vi "Illini Hyperloop GUI v5.0.vi"() -> ()   [LabVIEW 2015]
uses:
  <vilib>/robotics/Controls/Attitude Indicator/Attitude Indicator.xctl
panel:
  out "Numeric 3":u16
  out "volat":dbl
  out "vy":dbl
  out "X2 Sen Stat":u16 format="%b"
  out "X1 Sen Stat":u16 format="%b"
  out "Tape Count":dbl
  out "Optical":dbl
  out "Temp5":dbl
  out "Temp4":dbl
  out "Temp3":dbl
  out "Temp2":dbl
  out "Temp1":dbl
  out "Time Since Coast":dbl
  out "Time Since Accel":dbl
  out "PCB Current mA":dbl(slide) scale=0.0..200.0
  out "Voltage 2":dbl(slide) scale=0.0..17.0
  out "True Position":dbl
  out "Sensor Status Bits":u16 format="%b"
  out "Pressure Status":bool
  out "Temp Status":bool=TRUE
  out "Velocity Status":bool
  out "Position Status":bool
  out "Acceleration Status":bool
  out "Voltage Status":bool
  out "PCB Current Status":bool
  in  "Pod State":u16(ring) items=["Pod Startup", "Safety Setup", "Safe Mode", "Functional Test", "Launch Ready", "Accel", "Coast", "Brake"]
  out "X2 Online":bool
  out "X1 Online":bool
  out "X2 State":dbl
  out "X1 State":dbl
  out "Position Chart":dbl(graph)
  out "Brake Pressure":dbl
  out "RPM":dbl
  out "Accel 3":dbl
  out "Accel 2":dbl
  out "Accel 1":dbl
  out "True Accel":dbl
  out "True Velocity":dbl
  out "Pull Tab connected":bool
  out "Voltage 1":dbl(slide) scale=0.0..17.0
  out "Ride Height":cluster{u16, u16, u16}(graph)
  out "Y, Z Accel":cluster{u16, u16}(graph)
  out "Temp Chart":cluster{u16, u16, u16, u16, u16}(graph)
  out "Brake Pressure Chart":dbl(graph)
  out "Velocity chart":dbl(graph)
  out "Acceleration Chart":cluster{dbl, dbl, dbl, dbl}(graph)
  in  "Send Command Button":bool
  in  "Command to Send":T1(ring)
  in  "Connection Status":enum16{"Disconnected", "Connected"}(ring)
  out "Attitude Indicator":cluster{"Roll":dbl, "Pitch":dbl}(xcontrol)
  in  "EMERGENCY BRAKE":bool
  in  "Functional Test Tab Control":enum32{"Network / File Info", "Program Control"}(tab)
  out "Client Closed":string="The client VI closed the connection."
  in  "Connect to":string="192.168.137.100"
  in  "timeout ms":i32=1000
  in  "port":u16=8800
  in  "ms per loop":u32
  in  "bytes per write":i32=1000
  out "Base File Name":string
  in  "Stop Program":bool
  out "Producer Error Messages":errorcluster
  out "Consumer Error Messages":errorcluster
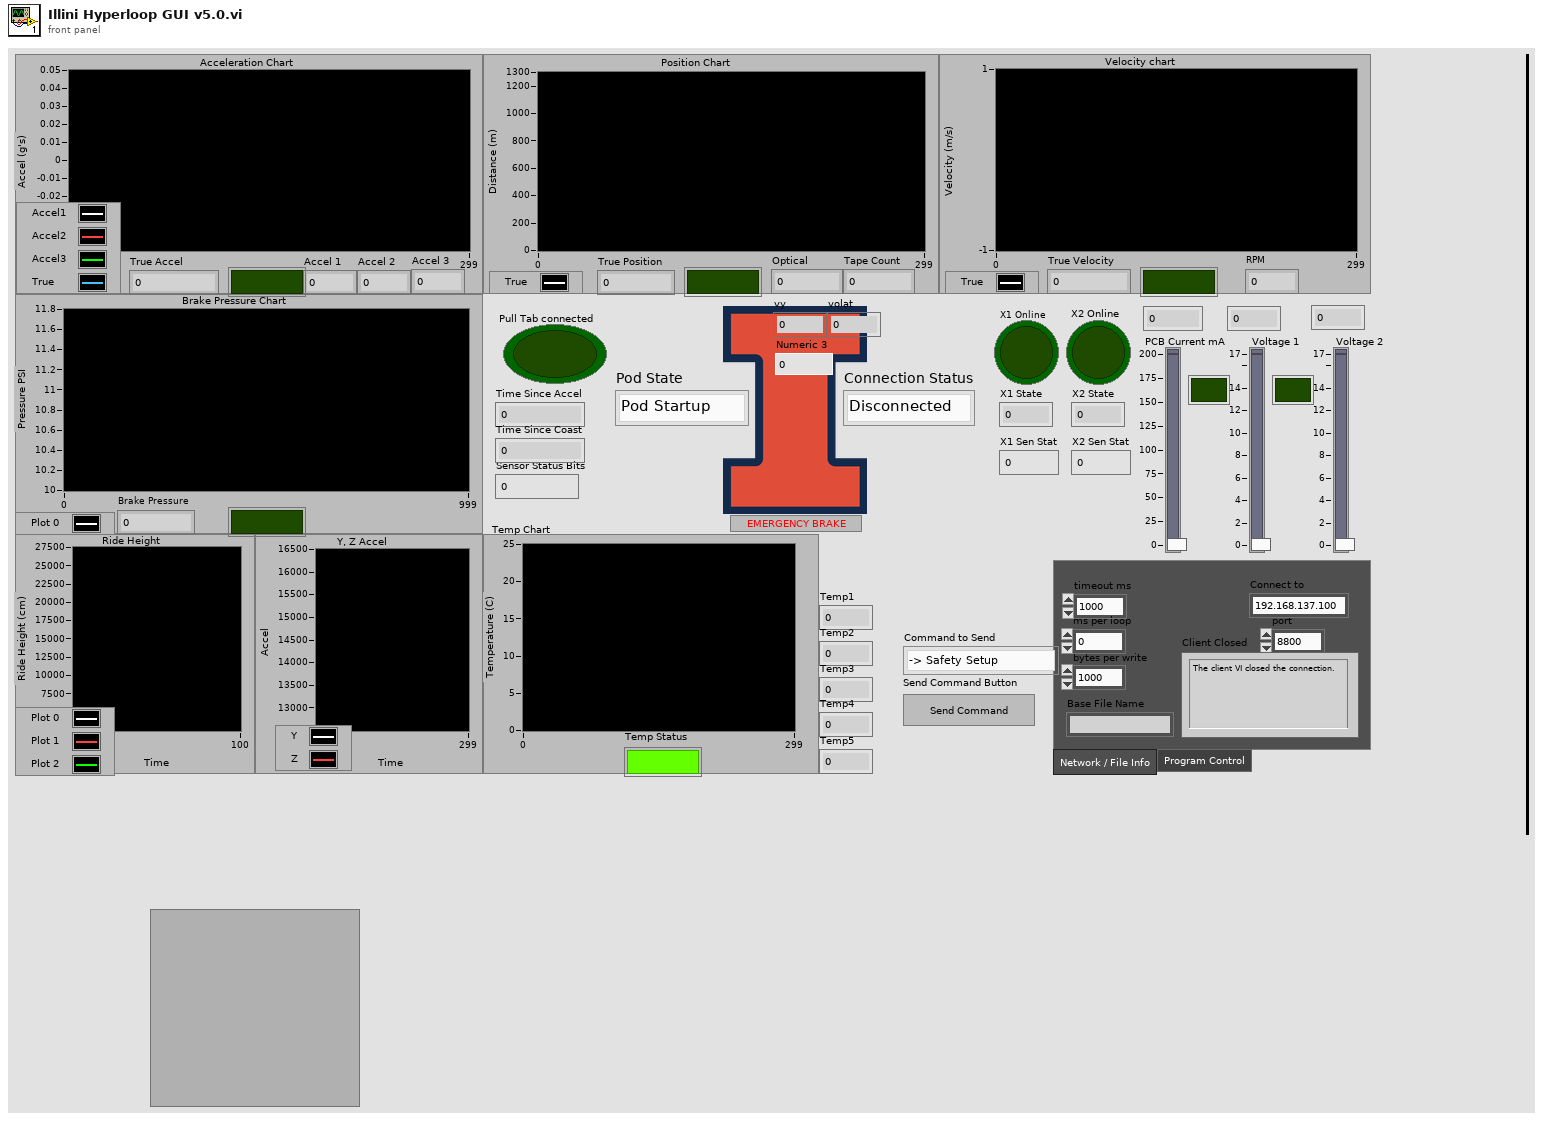
[diagram p1: front panel]
types:
  T1 = enum16{"-> Safety Setup", "-> Safe Mode", "-> Functional Test", "-> Ready to Launch", "-> Flight Brake", "EMERGENCY BRAKE", "Reset Sensors", "Calibrate Sensors", "Manual Brake ", "Manual Brake Reverse"}
  T2 = enum16{"Standard", "Buffered", "CRLF", "Immediate"}
  T3 = cluster{"Numeric 3":u16, "Numeric 3":u16, "Numeric 3":u16}
  T4 = cluster{"Accel 1":dbl, "Accel 2":dbl, "Accel 3":dbl, "True Accel":dbl}
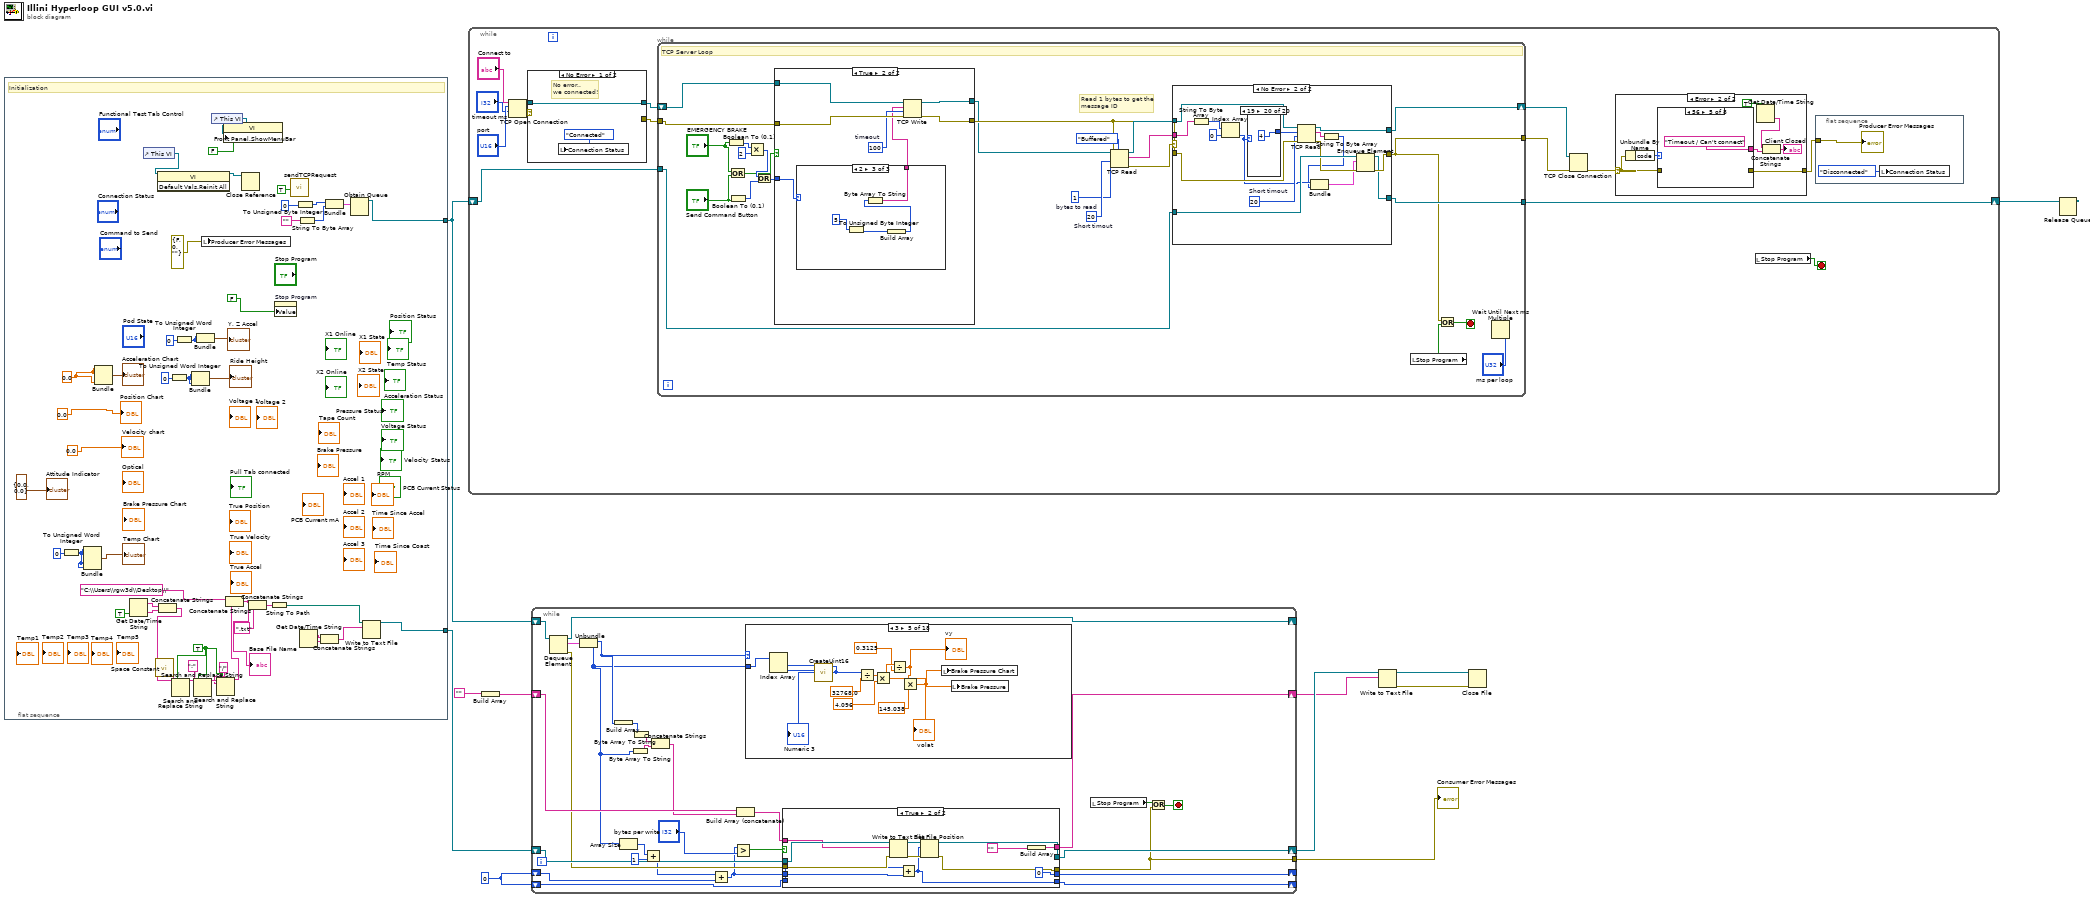
[diagram p0: block diagram]
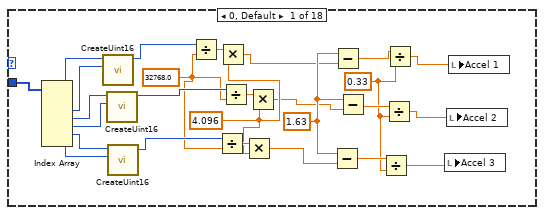
[diagram p2: hidden frame]
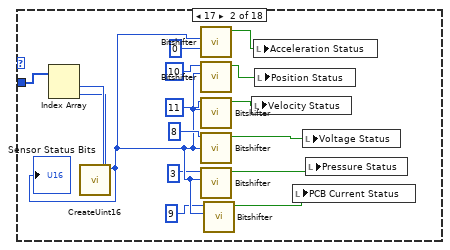
[diagram p3: hidden frame]
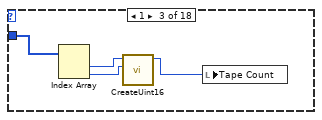
[diagram p4: hidden frame]
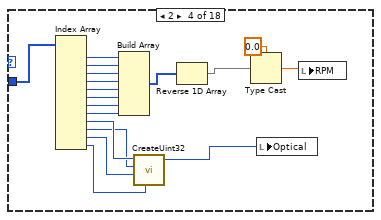
[diagram p5: hidden frame]
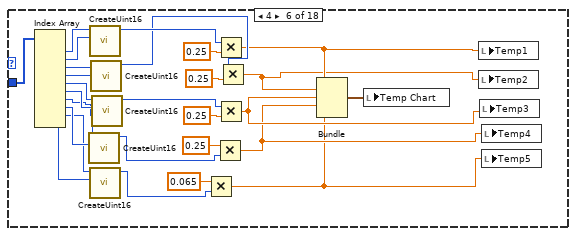
[diagram p6: hidden frame]
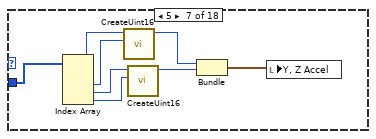
[diagram p7: hidden frame]
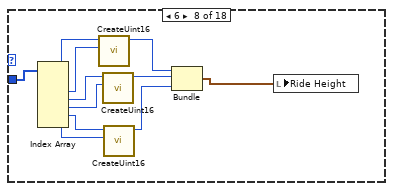
[diagram p8: hidden frame]
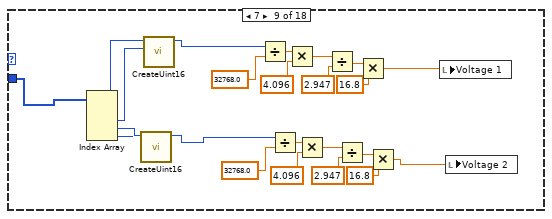
[diagram p9: hidden frame]
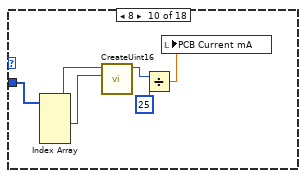
[diagram p10: hidden frame]
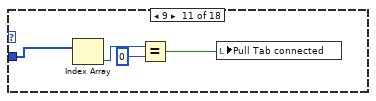
[diagram p11: hidden frame]
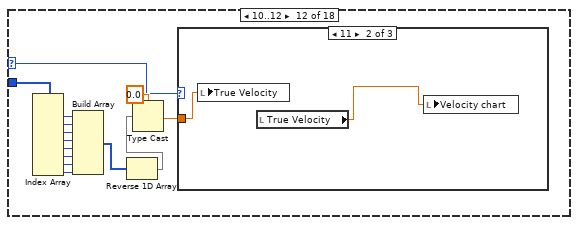
[diagram p12: hidden frame]
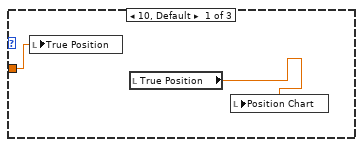
[diagram p13: hidden frame]
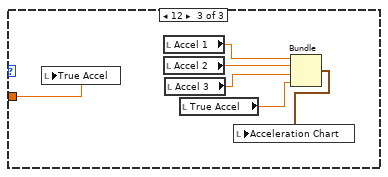
[diagram p14: hidden frame]
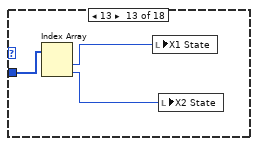
[diagram p15: hidden frame]
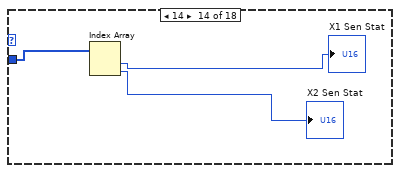
[diagram p16: hidden frame]
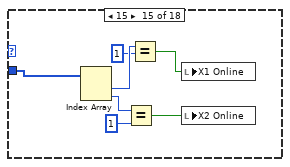
[diagram p17: hidden frame]
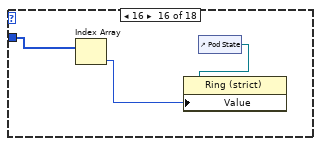
[diagram p18: hidden frame]
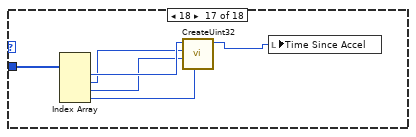
[diagram p19: hidden frame]
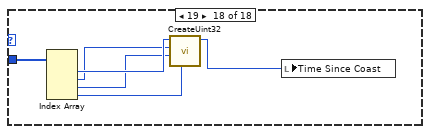
[diagram p20: hidden frame]
diagram:
  w2 = 0
  n1 = flat-sequence {
    tunnel: [w58] -> w11
    tunnel: [w46] -> w7
    frame #0 {
      w14 = 0.0
      w33 = TRUE ("want seconds? (F)")
      # "Initialization"
      n2 = To Unsigned Word Integer(number=0) -> (unsigned 16bit integer=w22:u16)
      n3 = Bundle(w22, w22, w22, w22, w22) -> (→"Temp Chart":cluster{u16, u16, u16, u16, u16})  [unwired: 1 in]
      n4 = Bundle(w14, w14, w14, w14) -> (→"Acceleration Chart":cluster{dbl, dbl, dbl, dbl})  [unwired: 1 in]
      n5 = Get Date/Time String(want seconds? (F)=TRUE) -> (date string=w44:string, time string=w43:string)  [unwired: 2 in]
      n6 = control-ref of="This VI"() -> (w51:refnum<vi>)
      n7 = call <vilib>:"Space Constant.vi"() -> ("String"=w45:string)
      n8 = invoke class="VI" method="Default Vals.Reinit All"(reference=w51) -> (reference out=w50:refnum<vi>)  [unwired: 2 in, 2 out]
      n9 = Concatenate Strings(w44, w43) -> (w42:string)
      n10 = To Unsigned Word Integer(number=0) -> (unsigned 16bit integer=w16:u16)
      n11 = Search and Replace String(replace all?=w33, input string=w42, search string=w45) -> (result string=w40:string)  [unwired: 5 in, 3 out]
      n12 = To Unsigned Word Integer(number=0) -> (unsigned 16bit integer=w19:u16)
      n13 = Bundle(w16, w16, w16) -> (→"Ride Height":cluster{u16, u16, u16})  [unwired: 1 in]
      n14 = Search and Replace String(replace all?=w33, input string=w40, search string=":" ("Functional Test 1 Data")) -> (result string=w36:string)  [unwired: 5 in, 3 out]
      n15 = Bundle(w19, w19) -> (→"Y, Z Accel":cluster{u16, u16})  [unwired: 1 in]
      n16 = local write "Producer Error Messages"(errorcluster {"status"=FALSE, "code"=0, "source"=""} ("error constant")) -> ()
      n17 = control-ref of="This VI"() -> (w55:refnum<vi>)
      n18 = Search and Replace String(replace all?=w33, input string=w36, search string="/" ("Functional Test 1 Data")) -> (result string=w35:string)  [unwired: 5 in, 3 out]
      n19 = property class="VI"(reference=w55, "Front Panel.ShowMenuBar"=FALSE ("Front Panel Window:Show Menu Bar")) -> ()  [unwired: 1 in, 2 out]
      n20 = Concatenate Strings("C:\\Users\\rgw3d\\Desktop\\" ("Functional Test 1 Data"), w35) -> (w31:string)
      "Base File Name" <- w31
      n21 = Close Reference(reference=w50) -> ()  [unwired: 1 in, 1 out]
      n22 = Concatenate Strings(w31, ".txt" ("Functional Test 1 Data")) -> (w32:string)
      n23 = String To Path(string=w32) -> (path=w37:path)
      n24 = property on="Stop Program" class="Bool (strict)"("Value"=FALSE) -> ()  [unwired: 2 in, 2 out]
      n25 = call "sendTCPRequest.vi"("Force Reset"=TRUE) -> ()  [unwired: 9 in, 2 out]
      n26 = To Unsigned Byte Integer(number=0) -> (unsigned 8bit integer=w28:u8)
      n27 = String To Byte Array(string="") -> (unsigned byte array=w26:u8[])
      n28 = Get Date/Time String() -> (date string=w49:string, time string=w48:string)  [unwired: 3 in]
      n29 = Concatenate Strings(w49, w48) -> (w47:string)
      n30 = Bundle(w28, "unsigned byte array"=w26) -> (w25:cluster{u8, "unsigned byte array":u8[]})  [unwired: 1 in]
      n31 = Obtain Queue(element data type=w25) -> (queue out=w58:refnum<queue>)  [unwired: 4 in, 2 out]
      n32 = Write to Text File(file (use dialog)=w37, text=w47) -> (refnum out=w46:refnum<file>)  [unwired: 2 in, 2 out]
      "Attitude Indicator" <- cluster{"Roll":dbl, "Pitch":dbl} {"Roll"=0.0, "Pitch"=0.0} ("Attitude Indicator")
      "Velocity chart" <- 0.0
      "Position Chart" <- 0.0
    }
  }
  n33 = while {
    shift-right: [w65] -> w1
    shift-left: w11 -> [w66]
    stop <- w62 stop-if-true
    n34 = TCP Open Connection(address="Connect to", remote port or service name="port", timeout ms (60000)="timeout ms") -> (connection ID=w67:refnum<k5>, error out=w68:errorcluster)  [unwired: 2 in]
    n35 = case shown="No Error" w68 {
      selector: w68 -> [_ w78]
      tunnel: w67 -> [w76 w79]
      tunnel: [w76 w79] -> w60
      tunnel: [_ w78] -> w59
      frame No Error {
        # "No error.. \nwe connected!"
        n36 = local write "Connection Status"(enum16{"Disconnected", "Connected"}."Connected" ("Connection Status")) -> ()
      }
      frame Error {
        n37 = local write "Connection Status"(enum16{"Disconnected", "Connected"}."Disconnected" ("Connection Status")) -> ()
      }
    }
    n38 = while {
      tunnel: w59 -> [w118]
      tunnel: [w98] -> w64
      tunnel: w66 -> [w102]
      tunnel: [w99] -> w65
      shift-right: [w97] -> w61
      shift-left: w60 -> [w119]
      stop <- w117 stop-if-true
      w107 = 1  # bytes to read
      w108 = 20  # Short timout
      # "Read 1 bytes to get the \nmessage ID"
      # "TCP Server Loop"
      n39 = Boolean To (0,1)(Boolean="EMERGENCY BRAKE") -> (0, 1=w113:i16)
      n40 = Or(x="EMERGENCY BRAKE", y="Send Command Button") -> (x .or. y?=w110:bool)
      n41 = Boolean To (0,1)(Boolean="Send Command Button") -> (0, 1=w114:i16)
      n42 = Multiply(x=w113, y=2) -> (x*y=w112:i32)
      n43 = Or(x=w112, y=w114) -> (x .or. y?=w111:i32)
      n44 = case shown="True" w110 {
        tunnel: w119 -> [w167 w174]
        tunnel: w118 -> [w166 w172]
        tunnel: [w166 w171] -> w101
        tunnel: [w167 w173] -> w100
        tunnel: w111 -> [_ w168]
        frame False {
        }
        frame True {
          w170 = 100  # timeout
          n45 = case shown="2" w168 {
            tunnel: ["" ("string") w177 w181] -> w169
            frame 0, Default {
            }
            frame 1 {
              n46 = control-ref of="Command to Send"() -> (w176:refnum<vi>)
              n47 = property class="Enum (strict)"(reference=w176) -> ("Value"=w179:T1)  [unwired: 1 in, 2 out]
              n48 = To Unsigned Byte Integer(number=w179) -> (unsigned 8bit integer=w180:u8)
              n49 = Build Array(w180) -> (w178:u8[])
              n50 = Byte Array To String(unsigned byte array=w178) -> (string=w177:string)
            }
            frame 2 {
              n51 = To Unsigned Byte Integer(number=5) -> (unsigned 8bit integer=w184:u8)
              n52 = Build Array(w184) -> (w182:u8[])
              n53 = Byte Array To String(unsigned byte array=w182) -> (string=w181:string)
            }
          }
          n54 = TCP Write(connection ID=w174, data in=w169, error in (no error)=w172, 9:w170) -> (connection ID out=w173:refnum<k5>, error out=w171:errorcluster)  [unwired: 1 out]
        }
      }
      n55 = TCP Read(connection ID=w100, bytes to read=w107, error in (no error)=w101, 7:T2."Buffered" ("mode (standard)"), 9:w108) -> (connection ID out=w105:refnum<k5>, data out=w104:string, error out=w106:errorcluster)
      n56 = case shown="No Error" w106 {
        selector: w106 -> [w125 _]
        tunnel: w101 -> [w126 w137]
        tunnel: [w124 w144] -> w98
        tunnel: w105 -> [w123 w139]
        tunnel: [w123 w138] -> w97
        tunnel: w104 -> [_ w142]
        tunnel: w102 -> [w122 w145]
        tunnel: [w122 w143] -> w99
        frame Error {
          # "If the error code is 56 (no data available to read - which will happen when we are reading faster than the beaglebone can send data) Then parse out the error. \nIf the error code is not 56, then we have a problem"
          n57 = Unbundle By Name(w125) -> ("code"=w127:i32)
          n58 = case shown="56" w127 {
            tunnel: w125 -> [w128 _]
            tunnel: [w128 w129] -> w124
            tunnel: w126 -> [_ w129]
            frame Default {
            }
            frame 56 {
            }
          }
        }
        frame No Error {
          w135 = 20  # Short timout
          n59 = String To Byte Array(string=w142) -> (unsigned byte array=w140:u8[])
          n60 = Index Array(array=w140, index=0) -> (element=w133:u8)
          n61 = case shown="19" w133 {
            tunnel: [6 2 12 2 10 4 6 4 4 1 8 ("index") 8 ("index") 8 ("index") 2 ("index") 2 ("index") 2 ("index") 1 ("index") 2 ("index") 4 ("index") 4 ("index")] -> w130
            frame 0, Default {
            }
            frame 1 {
            }
            frame 2 {
            }
            frame 3 {
            }
            frame 4 {
            }
            frame 5 {
            }
            frame 6 {
            }
            frame 7 {
            }
            frame 8 {
            }
            frame 9 {
            }
            frame 10 {
            }
            frame 11 {
            }
            frame 12 {
            }
            frame 13 {
            }
            frame 14 {
            }
            frame 15 {
            }
            frame 16 {
            }
            frame 17 {
            }
            frame 18 {
            }
            frame 19 {
            }
          }
          n62 = TCP Read(connection ID=w139, bytes to read=w130, error in (no error)=w137, 9:w135) -> (connection ID out=w138:refnum<k5>, data out=w132:string, error out=w136:errorcluster)  [unwired: 1 in]
          n63 = String To Byte Array(string=w132) -> (unsigned byte array=w131:u8[])
          n64 = Bundle(w133, "unsigned byte array"=w131) -> (w134:cluster{u8, "unsigned byte array":u8[]})  [unwired: 1 in]
          n65 = Enqueue Element(queue=w145, element=w134, error in (no error)=w136) -> (queue out=w143:refnum<queue>, error out=w144:errorcluster)  [unwired: 1 in, 1 out]
        }
      }
      n66 = local read "Stop Program"() -> (w121:bool)
      n67 = Or(x=w98, y=w121) -> (x .or. y?=w117:bool)
      n68 = Wait Until Next ms Multiple(millisecond multiple="ms per loop") -> ()  [unwired: 1 out]
    }
    n69 = TCP Close Connection(connection ID=w61, error in (no error)=w64) -> (error out=w72:errorcluster)  [unwired: 2 out]
    n70 = case shown="Error" w72 {
      selector: w72 -> [w80 w86]
      tunnel: [w80 w85] -> w71
      frame No Error {
      }
      frame Error {
        n71 = Unbundle By Name(w86) -> ("code"=w87:i32)
        n72 = case shown="56" w87 {
          tunnel: w86 -> [_ _ w91 _ _ _ _ _]
          tunnel: [_ _ w91 _ _ _ _ _] -> w85
          tunnel: ["The network is down, \nunreachable, or has been reset." "The specified network \naddress is currently in use." "Error" "The system caused the network \nconnection to be aborted." "Timeout / Can't connect" "Error 63. LabVIEW: The network connection \nwas refused by the server." "\tThe network connection\n is not yet established." "The network connection\n was closed by the peer."] -> w82
          frame 59 {
          }
          frame 60 {
          }
          frame Default {
          }
          frame 62 {
          }
          frame 56 {
          }
          frame 63 {
          }
          frame 64 {
          }
          frame 66 {
          }
        }
        n73 = Get Date/Time String(want seconds? (F)=TRUE) -> (time string=w83:string)  [unwired: 2 in, 1 out]
        n74 = Concatenate Strings(w83, w82) -> (→"Client Closed":string)
      }
    }
    n75 = local read "Stop Program"() -> (w62:bool)
    n76 = flat-sequence {
      tunnel: w71 -> [w74]
      frame #0 {
        n77 = local write "Connection Status"(enum16{"Disconnected", "Connected"}."Disconnected" ("Connection Status")) -> ()
        "Producer Error Messages" <- w74
      }
    }
  }
  n78 = Build Array("") -> (w8:string[])
  n79 = while {
    shift-right: [w212] -> _
    shift-left: w11 -> [w211]
    tunnel: [w201] -> w10
    shift-right: [w196] -> w3
    shift-left: w8 -> [w208]
    shift-right: [w206] -> w6
    shift-left: w7 -> [w207]
    shift-right: [w200] -> _
    shift-left: w2 -> [w204]
    shift-right: [w194] -> _
    shift-left: w2 -> [w195]
    stop <- w209 stop-if-true
    n80 = Dequeue Element(queue=w211) -> (queue out=w212:refnum<queue>, element=w205:cluster{u8, "unsigned byte array":u8[]}, error out=w203:errorcluster)  [unwired: 2 in, 1 out]
    n81 = Unbundle(w205) -> (w190:u8, "unsigned byte array"=w188:u8[])
    n82 = Build Array(w190) -> (w189:u8[])
    n83 = Array Size(array=w188) -> (size(s)=w193:i32)
    n84 = Byte Array To String(unsigned byte array=w188) -> (string=w187:string)
    n85 = Byte Array To String(unsigned byte array=w189) -> (string=w186:string)
    n86 = Add(x=w193, y=1) -> (x+y=w191:i32)
    n87 = Concatenate Strings(w186, w187) -> (w185:string)
    n88 = Add(x=w191, y=w204) -> (x+y=w197:i32)
    n89 = Greater?(x=w197, y="bytes per write") -> (0:w202:bool)
    n90 = Build Array (concatenate)(w208, w185) -> (w198:string[])
    n91 = case shown="3" w190 {
      selector: w190 -> [_ _ _ _ _ _ _ _ _ _ _ w371 _ _ _ _ _ _]
      tunnel: w188 -> [w238 w254 w258 w276 w288 w313 w317 w325 w353 w362 w367 w372 w394 w397 w404 w407 w413 w415]
      frame 0, Default {
        w220 = 0.33 ("y")
        w216 = 1.63 ("y")
        w225 = 4.096 ("y")
        w224 = 32768.0
        n92 = Index Array(array=w238) -> (element #1=w237:u8, element #2=w236:u8, element #3=w235:u8, element #4=w234:u8, element #5=w233:u8, element #6=w232:u8)  [unwired: 6 in]
        n93 = call "CreateUint16.vi"("high"=w236, "low"=w237) -> ("Numeric 3"=w231:u16)  [unwired: 9 in]
        n94 = call "CreateUint16.vi"("high"=w234, "low"=w235) -> ("Numeric 3"=w226:u16)  [unwired: 9 in]
        n95 = call "CreateUint16.vi"("high"=w232, "low"=w233) -> ("Numeric 3"=w227:u16)  [unwired: 9 in]
        n96 = Divide(x=w231, y=w224) -> (x/y=w230:dbl)
        n97 = Divide(x=w227, y=w224) -> (x/y=w228:dbl)
        n98 = Multiply(x=w230, y=w225) -> (x*y=w215:dbl)
        n99 = Divide(x=w226, y=w224) -> (x/y=w229:dbl)
        n100 = Multiply(x=w228, y=w225) -> (x*y=w213:dbl)
        n101 = Multiply(x=w229, y=w225) -> (x*y=w214:dbl)
        n102 = Subtract(x=w216, y=w213) -> (x-y=w221:dbl)
        n103 = Subtract(x=w216, y=w215) -> (x-y=w223:dbl)
        n104 = Subtract(x=w216, y=w214) -> (x-y=w222:dbl)
        n105 = Divide(x=w221, y=w220) -> (x/y=w219:dbl)
        n106 = Divide(x=w222, y=w220) -> (x/y=w218:dbl)
        n107 = Divide(x=w223, y=w220) -> (x/y=w217:dbl)
        n108 = local write "Accel 3"(w219) -> ()
        n109 = local write "Accel 2"(w218) -> ()
        n110 = local write "Accel 1"(w217) -> ()
      }
      frame 17 {
        n111 = Index Array(array=w254) -> (element #1=w253:u8, element #2=w252:u8)  [unwired: 2 in]
        n112 = call "CreateUint16.vi"("high"=w252, "low"=w253) -> ("Numeric 3"=w241:u16)  [unwired: 9 in]
        "Sensor Status Bits" <- w241
        n113 = call "Bitshifter.vi"("Bits"=w241, "Type"=0) -> ("Output"=w250:bool)  [unwired: 9 in]
        n114 = call "Bitshifter.vi"("Bits"=w241, "Type"=10) -> ("Output"=w249:bool)  [unwired: 9 in]
        n115 = call "Bitshifter.vi"("Bits"=w241, "Type"=11) -> ("Output"=w246:bool)  [unwired: 9 in]
        n116 = call "Bitshifter.vi"("Bits"=w241, "Type"=8) -> ("Output"=w244:bool)  [unwired: 9 in]
        n117 = call "Bitshifter.vi"("Bits"=w241, "Type"=3) -> ("Output"=w243:bool)  [unwired: 9 in]
        n118 = call "Bitshifter.vi"("Bits"=w241, "Type"=9) -> ("Output"=w242:bool)  [unwired: 9 in]
        n119 = local write "Velocity Status"(w246) -> ()
        n120 = local write "Acceleration Status"(w250) -> ()
        n121 = local write "Position Status"(w249) -> ()
        n122 = local write "PCB Current Status"(w242) -> ()
        n123 = local write "Voltage Status"(w244) -> ()
        n124 = local write "Pressure Status"(w243) -> ()
      }
      frame 1 {
        n125 = Index Array(array=w258) -> (element #1=w257:u8, element #2=w256:u8)  [unwired: 2 in]
        n126 = call "CreateUint16.vi"("high"=w256, "low"=w257) -> ("Numeric 3"=w255:u16)  [unwired: 9 in]
        n127 = local write "Tape Count"(w255) -> ()
      }
      frame 2 {
        n128 = Index Array(array=w276) -> (element #1=w269:u8, element #2=w268:u8, element #3=w267:u8, element #4=w266:u8, element #5=w265:u8, element #6=w264:u8, element #7=w263:u8, element #8=w262:u8, element #9=w275:u8, element #10=w274:u8, element #11=w273:u8, element #12=w272:u8)  [unwired: 12 in]
        n129 = Build Array(w269, w268, w267, w266, w265, w264, w263, w262) -> (w260:u8[])
        n130 = call "CreateUint32.vi"("Numeric in"=w272, "Numeric 3"=w273, "Numeric 4"=w274, "Numeric 5"=w275) -> ("Numeric out"=w271:u32)  [unwired: 7 in]
        n131 = Reverse 1D Array(array=w260) -> (reversed array=w259:u8[])
        n132 = Type Cast(type=0.0, x=w259) -> (*(type *) &x=w261:dbl)
        n133 = local write "Optical"(w271) -> ()
        n134 = local write "RPM"(w261) -> ()
      }
      frame 3 {
        n135 = Index Array(array=w288) -> (element #1=w287:u8, element #2=w286:u8)  [unwired: 2 in]
        n136 = call "CreateUint16.vi"("high"=w286, "low"=w287) -> ("Numeric 3"=w283:u16)  [unwired: 9 in]
        "Numeric 3" <- w283
        n137 = Divide(x=w283, y=32768.0) -> (x/y=w285:dbl)
        n138 = Multiply(x=w285, y=4.096) -> (x*y=w279:dbl)
        "volat" <- w279
        n139 = Divide(x=w279, y=0.3125) -> (x/y=w277:dbl)
        "vy" <- w277
        n140 = Multiply(x=w277, y=145.038) -> (x*y=w280:dbl)
        n141 = local write "Brake Pressure Chart"(w280) -> ()
        n142 = local write "Brake Pressure"(w280) -> ()
      }
      frame 4 {
        n143 = Index Array(array=w313) -> (element #1=w315:u8, element #2=w314:u8, element #3=w312:u8, element #4=w311:u8, element #5=w310:u8, element #6=w309:u8, element #7=w308:u8, element #8=w307:u8, element #9=w306:u8, element #10=w305:u8)  [unwired: 10 in]
        n144 = call "CreateUint16.vi"("high"=w307, "low"=w308) -> ("Numeric 3"=w296:u16)  [unwired: 9 in]
        n145 = call "CreateUint16.vi"("high"=w314, "low"=w315) -> ("Numeric 3"=w302:u16)  [unwired: 9 in]
        n146 = call "CreateUint16.vi"("high"=w305, "low"=w306) -> ("Numeric 3"=w294:u16)  [unwired: 9 in]
        n147 = call "CreateUint16.vi"("high"=w311, "low"=w312) -> ("Numeric 3"=w301:u16)  [unwired: 9 in]
        n148 = call "CreateUint16.vi"("high"=w309, "low"=w310) -> ("Numeric 3"=w297:u16)  [unwired: 9 in]
        n149 = Multiply(x=0.065 ("y"), y=w294) -> (x*y=w289:dbl)
        n150 = Multiply(x=0.25 ("y"), y=w296) -> (x*y=w290:dbl)
        n151 = Multiply(x=w302, y=0.25) -> (x*y=w293:dbl)
        n152 = Multiply(x=w297, y=0.25) -> (x*y=w291:dbl)
        n153 = Multiply(x=w301, y=0.25) -> (x*y=w292:dbl)
        n154 = Bundle(w293, w292, w291, w290, w289) -> (w304:cluster{dbl, dbl, dbl, dbl, dbl})  [unwired: 1 in]
        n155 = local write "Temp Chart"(w304) -> ()
        n156 = local write "Temp1"(w293) -> ()
        n157 = local write "Temp2"(w292) -> ()
        n158 = local write "Temp3"(w291) -> ()
        n159 = local write "Temp4"(w290) -> ()
        n160 = local write "Temp5"(w289) -> ()
      }
      frame 5 {
        n161 = Index Array(array=w317) -> (element #1=w322:u8, element #2=w321:u8, element #3=w320:u8, element #4=w319:u8)  [unwired: 4 in]
        n162 = call "CreateUint16.vi"("high"=w321, "low"=w322) -> ("Numeric 3"=w323:u16)  [unwired: 9 in]
        n163 = call "CreateUint16.vi"("high"=w319, "low"=w320) -> ("Numeric 3"=w318:u16)  [unwired: 9 in]
        n164 = Bundle("Numeric 3"=w323, "Numeric 3"=w318) -> (w316:cluster{"Numeric 3":u16, "Numeric 3":u16})  [unwired: 1 in]
        n165 = local write "Y, Z Accel"(w316) -> ()
      }
      frame 6 {
        n166 = Index Array(array=w325) -> (element #1=w333:u8, element #2=w332:u8, element #3=w331:u8, element #4=w330:u8, element #5=w329:u8, element #6=w328:u8)  [unwired: 6 in]
        n167 = call "CreateUint16.vi"("high"=w332, "low"=w333) -> ("Numeric 3"=w334:u16)  [unwired: 9 in]
        n168 = call "CreateUint16.vi"("high"=w330, "low"=w331) -> ("Numeric 3"=w327:u16)  [unwired: 9 in]
        n169 = call "CreateUint16.vi"("high"=w328, "low"=w329) -> ("Numeric 3"=w326:u16)  [unwired: 9 in]
        n170 = Bundle("Numeric 3"=w334, "Numeric 3"=w327, "Numeric 3"=w326) -> (w324:T3)  [unwired: 1 in]
        n171 = local write "Ride Height"(w324) -> ()
      }
      frame 7 {
        n172 = Index Array(array=w353) -> (element #1=w357:u8, element #2=w356:u8, element #3=w355:u8, element #4=w354:u8)  [unwired: 4 in]
        n173 = call "CreateUint16.vi"("high"=w354, "low"=w355) -> ("Numeric 3"=w337:u16)  [unwired: 9 in]
        n174 = call "CreateUint16.vi"("high"=w356, "low"=w357) -> ("Numeric 3"=w351:u16)  [unwired: 9 in]
        n175 = Divide(x=w351, y=32768.0) -> (x/y=w352:dbl)
        n176 = Divide(x=w337, y=32768.0) -> (x/y=w344:dbl)
        n177 = Multiply(x=w352, y=4.096) -> (x*y=w348:dbl)
        n178 = Multiply(x=w344, y=4.096) -> (x*y=w341:dbl)
        n179 = Divide(x=w348, y=2.947) -> (x/y=w346:dbl)
        n180 = Divide(x=w341, y=2.947) -> (x/y=w339:dbl)
        n181 = Multiply(x=w346, y=16.8) -> (x*y=w336:dbl)
        n182 = Multiply(x=w339, y=16.8) -> (x*y=w335:dbl)
        n183 = local write "Voltage 1"(w336) -> ()
        n184 = local write "Voltage 2"(w335) -> ()
      }
      frame 8 {
        n185 = Index Array(array=w362) -> (element #1=w361:u8, element #2=w363:u8)  [unwired: 4 in, 2 out]
        n186 = call "CreateUint16.vi"("high"=w363, "low"=w361) -> ("Numeric 3"=w360:u16)  [unwired: 9 in]
        n187 = Divide(x=w360, y=u16 25) -> (x/y=w358:dbl)
        n188 = local write "PCB Current mA"(w358) -> ()
      }
      frame 9 {
        n189 = Index Array(array=w367) -> (element=w366:u8)  [unwired: 1 in]
        n190 = Equal?(x=w366, y=u8 0) -> (x = y?=w364:bool)
        n191 = local write "Pull Tab connected"(w364) -> ()
      }
      frame 10..12 {
        n192 = Index Array(array=w372) -> (element #1=w380:u8, element #2=w379:u8, element #3=w378:u8, element #4=w377:u8, element #5=w376:u8, element #6=w375:u8, element #7=w374:u8, element #8=w373:u8)  [unwired: 8 in]
        n193 = Build Array(w380, w379, w378, w377, w376, w375, w374, w373) -> (w369:u8[])
        n194 = Reverse 1D Array(array=w369) -> (reversed array=w368:u8[])
        n195 = Type Cast(type=0.0, x=w368) -> (*(type *) &x=w370:dbl)
        n196 = case shown="11" w371 {
          tunnel: w370 -> [w383 w385 w391]
          frame 10, Default {
            n197 = local write "True Position"(w383) -> ()
            n198 = local read "True Position"() -> (w382:dbl)
            n199 = local write "Position Chart"(w382) -> ()
          }
          frame 11 {
            n200 = local write "True Velocity"(w385) -> ()
            n201 = local read "True Velocity"() -> (w384:dbl)
            n202 = local write "Velocity chart"(w384) -> ()
          }
          frame 12 {
            n203 = local write "True Accel"(w391) -> ()
            n204 = local read "Accel 1"() -> (w390:dbl)
            n205 = local read "Accel 2"() -> (w389:dbl)
            n206 = local read "Accel 3"() -> (w388:dbl)
            n207 = local read "True Accel"() -> (w387:dbl)
            n208 = Bundle("Accel 1"=w390, "Accel 2"=w389, "Accel 3"=w388, "True Accel"=w387) -> (w386:T4)  [unwired: 1 in]
            n209 = local write "Acceleration Chart"(w386) -> ()
          }
        }
      }
      frame 13 {
        n210 = Index Array(array=w394) -> (element #1=w393:u8, element #2=w392:u8)  [unwired: 2 in]
        n211 = local write "X1 State"(w393) -> ()
        n212 = local write "X2 State"(w392) -> ()
      }
      frame 14 {
        n213 = Index Array(array=w397) -> (element #1=→"X1 Sen Stat":u8, element #2=→"X2 Sen Stat":u8)  [unwired: 2 in]
      }
      frame 15 {
        n214 = Index Array(array=w404) -> (element #1=w403:u8, element #2=w401:u8)  [unwired: 2 in]
        n215 = Equal?(x=w401, y=u8 1) -> (x = y?=w399:bool)
        n216 = Equal?(x=w403, y=u8 1) -> (x = y?=w398:bool)
        n217 = local write "X1 Online"(w398) -> ()
        n218 = local write "X2 Online"(w399) -> ()
      }
      frame 16 {
        n219 = Index Array(array=w407) -> (element=w405:u8)  [unwired: 1 in]
        n220 = control-ref of="Pod State"() -> (w406:refnum<vi>)
        n221 = property class="Ring (strict)"(reference=w406, "Value"=w405) -> ()  [unwired: 1 in, 2 out]
      }
      frame 18 {
        n222 = Index Array(array=w413) -> (element #1=w412:u8, element #2=w411:u8, element #3=w410:u8, element #4=w409:u8)  [unwired: 4 in]
        n223 = call "CreateUint32.vi"("Numeric in"=w409, "Numeric 3"=w410, "Numeric 4"=w411, "Numeric 5"=w412) -> ("Numeric out"=w408:u32)  [unwired: 7 in]
        n224 = local write "Time Since Accel"(w408) -> ()
      }
      frame 19 {
        n225 = Index Array(array=w415) -> (element #1=w419:u8, element #2=w418:u8, element #3=w417:u8, element #4=w416:u8)  [unwired: 4 in]
        n226 = call "CreateUint32.vi"("Numeric in"=w416, "Numeric 3"=w417, "Numeric 4"=w418, "Numeric 5"=w419) -> ("Numeric out"=w414:u32)  [unwired: 7 in]
        n227 = local write "Time Since Coast"(w414) -> ()
      }
    }
    n228 = case shown="True" w202 {
      tunnel: w198 -> [w421 w428]
      tunnel: w207 -> [w424 w437]
      tunnel: [w424 w431] -> w206
      tunnel: w197 -> [w423 w426]
      tunnel: [w422 w434] -> w201
      tunnel: w203 -> [w422 w433]
      tunnel: [w423 0] -> w200
      tunnel: [w421 w429] -> w196
      tunnel: w195 -> [w420 w427]
      tunnel: [w420 w425] -> w194
      frame False {
      }
      frame True {
        n229 = Write to Text File(file (use dialog)=w437, text=w428, error in=w433) -> (refnum out=w436:refnum<file>, error out=w435:errorcluster)  [unwired: 1 in, 1 out]
        n230 = Add(x=w427, y=w426) -> (x+y=w425:i32)
        n231 = Set File Position(offset (in bytes) (0)=w425, refnum=w436, error in=w435) -> (refnum out=w431:refnum<file>, error out=w434:errorcluster)  [unwired: 1 in]
        n232 = Build Array("") -> (w429:string[])
      }
    }
    n233 = local read "Stop Program"() -> (w210:bool)
    n234 = Or(x=w210, y=w201) -> (x .or. y?=w209:bool)
  }
  "Consumer Error Messages" <- w10
  n235 = Write to Text File(file (use dialog)=w6, text=w3) -> (refnum out=w4:refnum<file>, error out=w5:errorcluster)  [unwired: 2 in, 1 out]
  n236 = Close File(refnum=w4, error in=w5) -> ()  [unwired: 2 out]
  n237 = Release Queue(queue=w1) -> ()  [unwired: 2 in, 3 out]
